vi "DrivePropertiesConvert.vi"(4 "Position Offset In":dbl, 5 "Channel Properties In":T2={"Channel Name"="", "Vel. Default"=5.0, "Acc. Default"=5.0, "Vel. Max"=5.0, "Vel. Min"=5.0, "Acc. Max"=5.0, "Acc. Min"=5.0, "Pulses/unit"=0.0, "Address"=0, "Pulse Offset"=0, "Pos Tolerance"=0.0, "Pulses/rev"=0.0, "Backlash/Eng units"=0.0, "Current Pos"=0.0, "Ch Status"=enum."Active", "Port Name"="", "Axis Transform mode"="", "Metadata Ch Name"="", "Type"=enum."MCode", "De Power Motor"=enum."FALSE", "ConfigString"=""} {"Current Pos" format="%.2f"; "Backlash/Eng units" format="%.2f"; "Pulses/rev" format="%.2f"; "Pos Tolerance" format="%.2f"; "Pulses/unit" format="%.2f"; "Acc. Min" format="%.2f"; "Acc. Max" format="%.2f"; "Vel. Min" format="%.2f"; "Vel. Max" format="%.2f"; "Acc. Default" format="%.2f"; "Vel. Default" format="%.2f"}, 6 "String in":string[](array[string]), 7 "Ch names In":string[](array[string]), 8 "Mode":enum16{"Cluster to String", "String to Cluster"}(ring)) -> (0 "Channel Properties Out":T2={"Channel Name"="", "Vel. Default"=5.0, "Acc. Default"=5.0, "Vel. Max"=5.0, "Vel. Min"=5.0, "Acc. Max"=5.0, "Acc. Min"=5.0, "Pulses/unit"=0.0, "Address"=0, "Pulse Offset"=0, "Pos Tolerance"=0.0, "Pulses/rev"=0.0, "Backlash/Eng units"=0.0, "Current Pos"=0.0, "Ch Status"=enum."Active", "Port Name"="", "Axis Transform mode"="", "Metadata Ch Name"="", "Type"=enum."MCode", "De Power Motor"=enum."FALSE", "ConfigString"=""} {"Current Pos" format="%.2f"; "Backlash/Eng units" format="%.2f"; "Pulses/rev" format="%.2f"; "Pos Tolerance" format="%.2f"; "Pulses/unit" format="%.2f"; "Acc. Min" format="%.2f"; "Acc. Max" format="%.2f"; "Vel. Min" format="%.2f"; "Vel. Max" format="%.2f"; "Acc. Default" format="%.2f"; "Vel. Default" format="%.2f"}, 1 "String Values":string[](array[string]), 2 "Ch names":string[](array[string]), 3 "Position Offset Out":dbl)   [LabVIEW 2022 SP3]
uses:
  DriveProperties.ctl
  Traverse Type.ctl
panel:
  in  "Type":T1
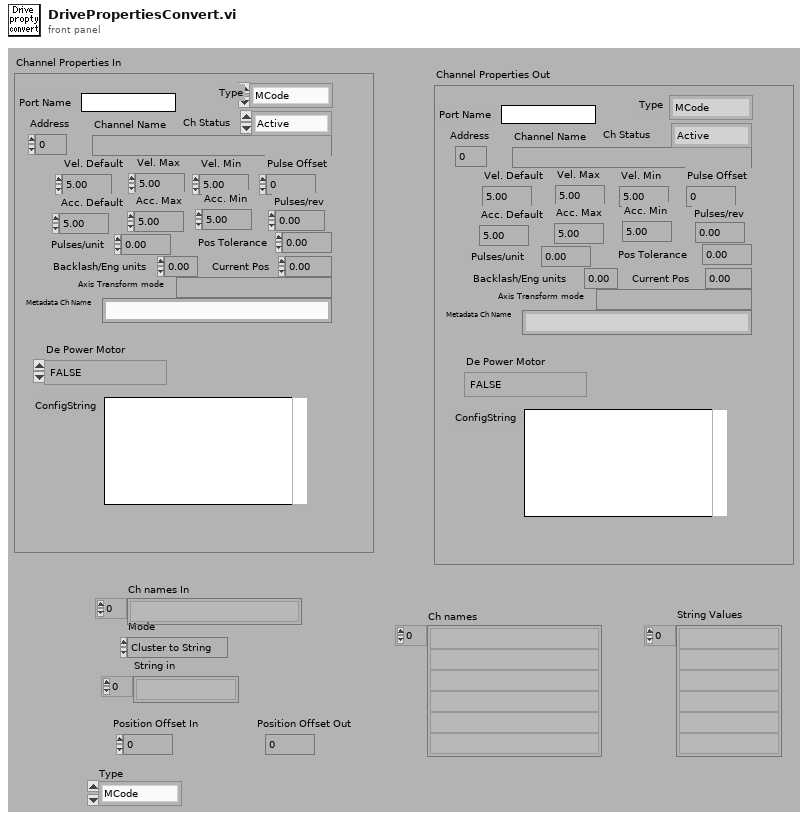
[diagram p1: front panel]
types:
  T1 = typedef "Traverse Type.ctl" = enum16{"MCode", "Dynamixel"}
  T2 = typedef "DriveProperties.ctl" = cluster{"Channel Name":string, "Vel. Default":sgl, "Acc. Default":sgl, "Vel. Max":sgl, "Vel. Min":sgl, "Acc. Max":sgl, "Acc. Min":sgl, "Pulses/unit":sgl, "Address":u8, "Pulse Offset":i32, "Pos Tolerance":sgl, "Pulses/rev":sgl, "Backlash/Eng units":sgl, "Current Pos":sgl, "Ch Status":enum16{"Active", "Offline", "Simulate"}, "Port Name":string, "Axis Transform mode":string, "Metadata Ch Name":string, "Type":T1, "De Power Motor":enum16{"TRUE", "FALSE"}, "ConfigString":string}
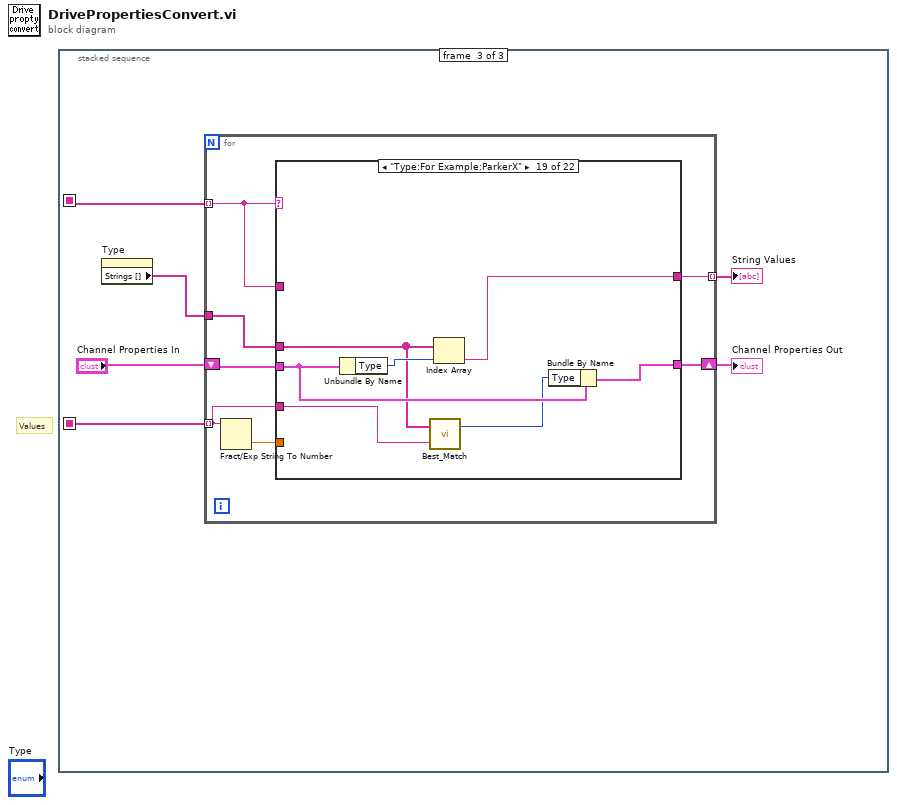
[diagram p0: block diagram]
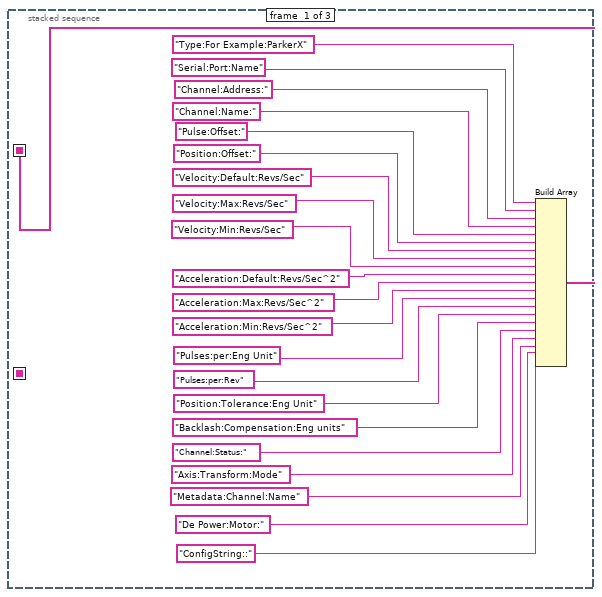
[diagram p2: hidden frame]
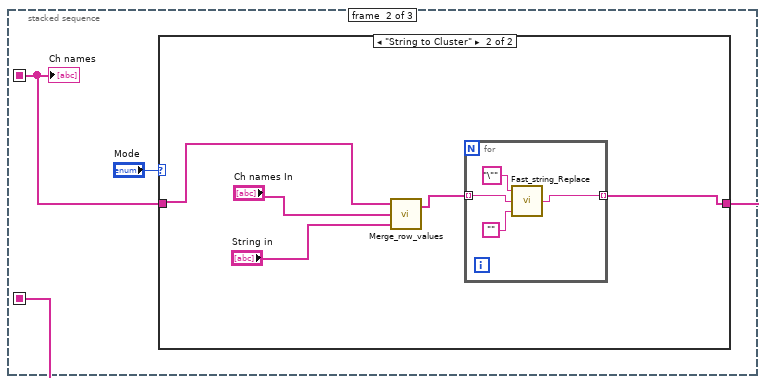
[diagram p3: hidden frame]
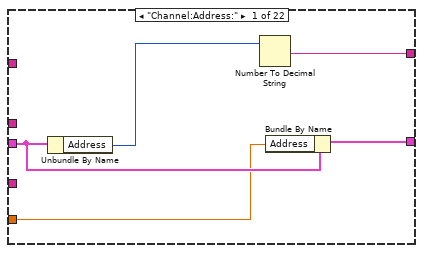
[diagram p5: hidden frame]
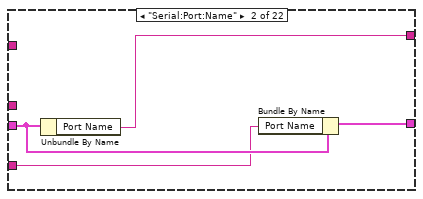
[diagram p6: hidden frame]
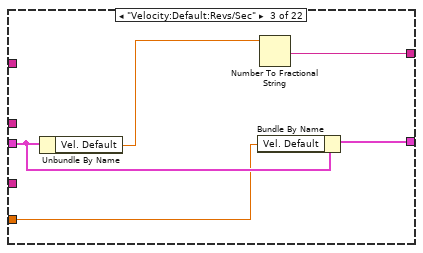
[diagram p7: hidden frame]
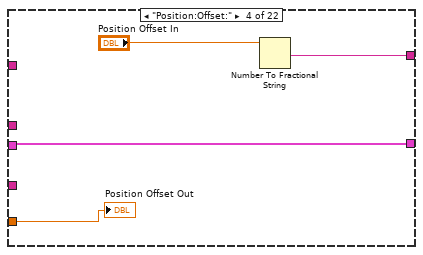
[diagram p8: hidden frame]
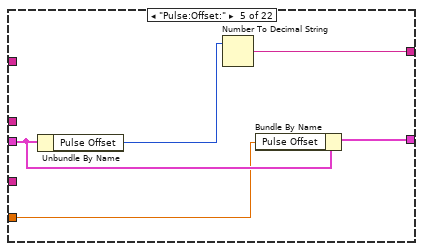
[diagram p9: hidden frame]
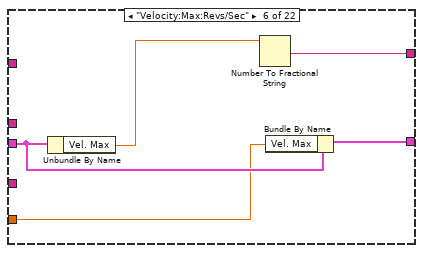
[diagram p10: hidden frame]
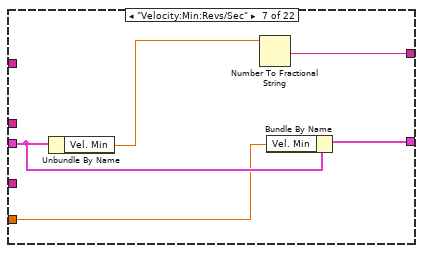
[diagram p11: hidden frame]
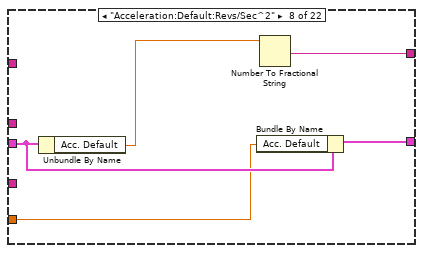
[diagram p12: hidden frame]
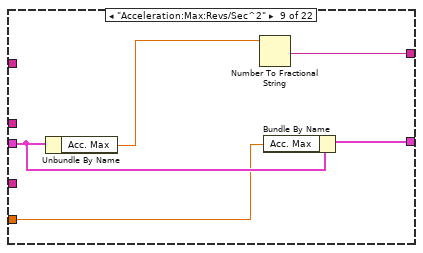
[diagram p13: hidden frame]
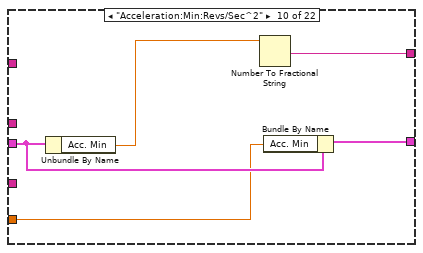
[diagram p14: hidden frame]
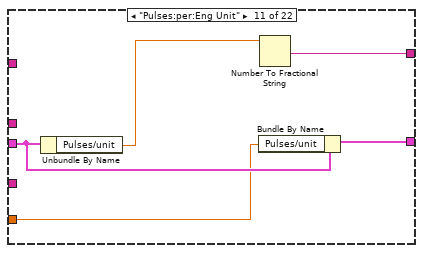
[diagram p15: hidden frame]
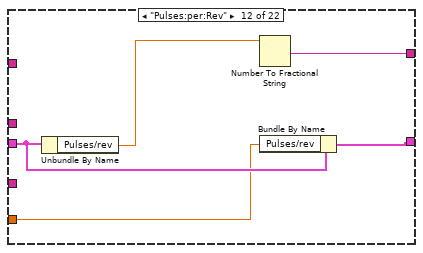
[diagram p16: hidden frame]
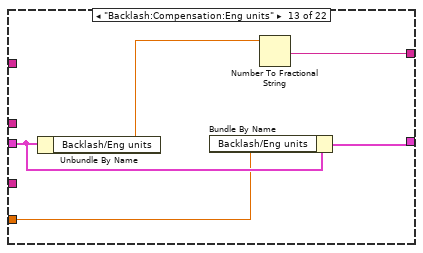
[diagram p17: hidden frame]
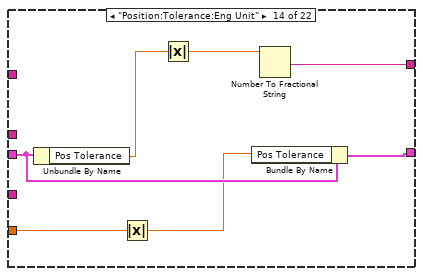
[diagram p18: hidden frame]
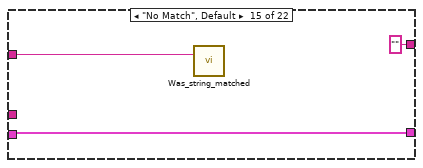
[diagram p19: hidden frame]
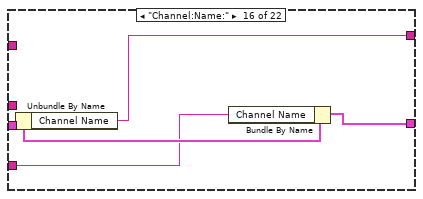
[diagram p20: hidden frame]
diagram:
  # "Values"
  n1 = stacked-sequence {
    seq-local: [w13 _ _] -> [_ w24 w41]
    seq-local: [_ w23 _] -> [_ _ w40]
    frame #0 {
      n2 = Build Array("Type:For Example:ParkerX", "Serial:Port:Name", "Channel:Address:", "Channel:Name:", "Pulse:Offset:", "Position:Offset:", "Velocity:Default:Revs/Sec", "Velocity:Max:Revs/Sec", "Velocity:Min:Revs/Sec", "Acceleration:Default:Revs/Sec^2", "Acceleration:Max:Revs/Sec^2", "Acceleration:Min:Revs/Sec^2", "Pulses:per:Eng Unit", "Pulses:per:Rev", "Position:Tolerance:Eng Unit", "Backlash:Compensation:Eng units", "Channel:Status:", "Axis:Transform:Mode", "Metadata:Channel:Name", "De Power:Motor:", "ConfigString::") -> (w13:string[])
    }
    frame #1 {
      n3 = case shown="\"String to Cluster\"" "Mode" {
        tunnel: [w26 w27] -> w23
        tunnel: w24 -> [w26 w29]
        frame "Cluster to String" {
        }
        frame "String to Cluster" {
          n4 = call "Merge_row_values.vi"("Present Row values"="String in", "Present Channels"="Ch names In", "Desired Channels"=w29) -> ("Desired Row values"=w28:string[])  [unwired: 1 out]
          n5 = for {
            tunnel: w28 -> [w35] mode=indexing
            tunnel: [w34] -> w27 mode=indexing
            n6 = call "Fast_string_Replace.vi"("Replace match with:"="", "Input String"=w35, "matchThis"="\"" ("regular expression")) -> ("Output String"=w34:string)  [unwired: 1 in, 1 out]
          }
        }
      }
      "Ch names" <- w24
    }
    frame #2 {
      n7 = property on="Type" class="Enum (strict)"() -> ("Strings []"=w36:string[])  [unwired: 2 in, 2 out]
      n8 = for {
        tunnel: w41 -> [w45] mode=indexing
        tunnel: w40 -> [w48] mode=indexing
        tunnel: [w46] -> w39 mode=indexing
        shift-right: [w43] -> w37
        shift-left: "Channel Properties In" -> [w44]
        tunnel: w36 -> [w42]
        n9 = Fract/Exp String To Number(string=w48) -> (number=w47:dbl)  [unwired: 4 out]
        n10 = case shown="\"Type:For Example:ParkerX\"" w45 {
          tunnel: w44 -> [w53 w57 w62 w64 w71 w76 w81 w86 w91 w96 w101 w106 w111 w118 w119 w124 w128 w132 w140 w146 w161 w171]
          tunnel: w48 -> [_ w55 _ _ _ _ _ _ _ _ _ _ _ _ _ w123 w127 w131 w136 w142 w157 w166]
          tunnel: [w50 w56 w59 w66 w67 w73 w78 w83 w88 w93 w98 w103 w108 w115 "" ("Channel Name") w125 w129 w133 w137 w143 w155 w168] -> w46
          tunnel: w47 -> [w52 _ w61 w63 w70 w75 w80 w85 w90 w95 w100 w105 w110 w117 _ _ _ _ _ _ _ _]
          tunnel: w45 -> [_ _ _ _ _ _ _ _ _ _ _ _ _ _ w120 _ _ _ _ _ _ _]
          tunnel: [w49 w54 w58 w64 w69 w72 w77 w82 w87 w92 w97 w102 w107 w112 w119 w122 w126 w130 w139 w145 w160 w170] -> w43
          tunnel: w42 -> [_ _ _ _ _ _ _ _ _ _ _ _ _ _ _ _ _ _ w135 _ _ _]
          frame "Channel:Address:" {
            n11 = Unbundle By Name(w53) -> ("Address"=w51:u8)
            n12 = Number To Decimal String(number=w51) -> (decimal integer string=w50:string)  [unwired: 1 out]
            n13 = Bundle By Name(cluster=w53, "Address"=w52) -> (w49:T2)
          }
          frame "Serial:Port:Name" {
            n14 = Unbundle By Name(w57) -> ("Port Name"=w56:string)
            n15 = Bundle By Name(cluster=w57, "Port Name"=w55) -> (w54:T2)
          }
          frame "Velocity:Default:Revs/Sec" {
            n16 = Unbundle By Name(w62) -> ("Vel. Default"=w60:sgl)
            n17 = Bundle By Name(cluster=w62, "Vel. Default"=w61) -> (w58:T2)
            n18 = Number To Fractional String(number=w60) -> (F-format string=w59:string)  [unwired: 3 out]
          }
          frame "Position:Offset:" {
            n19 = Number To Fractional String(number="Position Offset In") -> (F-format string=w66:string)  [unwired: 3 out]
            "Position Offset Out" <- w63
          }
          frame "Pulse:Offset:" {
            n20 = Unbundle By Name(w71) -> ("Pulse Offset"=w68:i32)
            n21 = Number To Decimal String(number=w68) -> (decimal integer string=w67:string)  [unwired: 1 out]
            n22 = Bundle By Name(cluster=w71, "Pulse Offset"=w70) -> (w69:T2)
          }
          frame "Velocity:Max:Revs/Sec" {
            n23 = Unbundle By Name(w76) -> ("Vel. Max"=w74:sgl)
            n24 = Number To Fractional String(number=w74) -> (F-format string=w73:string)  [unwired: 3 out]
            n25 = Bundle By Name(cluster=w76, "Vel. Max"=w75) -> (w72:T2)
          }
          frame "Velocity:Min:Revs/Sec" {
            n26 = Unbundle By Name(w81) -> ("Vel. Min"=w79:sgl)
            n27 = Number To Fractional String(number=w79) -> (F-format string=w78:string)  [unwired: 3 out]
            n28 = Bundle By Name(cluster=w81, "Vel. Min"=w80) -> (w77:T2)
          }
          frame "Acceleration:Default:Revs/Sec^2" {
            n29 = Unbundle By Name(w86) -> ("Acc. Default"=w84:sgl)
            n30 = Bundle By Name(cluster=w86, "Acc. Default"=w85) -> (w82:T2)
            n31 = Number To Fractional String(number=w84) -> (F-format string=w83:string)  [unwired: 3 out]
          }
          frame "Acceleration:Max:Revs/Sec^2" {
            n32 = Unbundle By Name(w91) -> ("Acc. Max"=w89:sgl)
            n33 = Number To Fractional String(number=w89) -> (F-format string=w88:string)  [unwired: 3 out]
            n34 = Bundle By Name(cluster=w91, "Acc. Max"=w90) -> (w87:T2)
          }
          frame "Acceleration:Min:Revs/Sec^2" {
            n35 = Unbundle By Name(w96) -> ("Acc. Min"=w94:sgl)
            n36 = Number To Fractional String(number=w94) -> (F-format string=w93:string)  [unwired: 3 out]
            n37 = Bundle By Name(cluster=w96, "Acc. Min"=w95) -> (w92:T2)
          }
          frame "Pulses:per:Eng Unit" {
            n38 = Unbundle By Name(w101) -> ("Pulses/unit"=w99:sgl)
            n39 = Bundle By Name(cluster=w101, "Pulses/unit"=w100) -> (w97:T2)
            n40 = Number To Fractional String(number=w99) -> (F-format string=w98:string)  [unwired: 3 out]
          }
          frame "Pulses:per:Rev" {
            n41 = Unbundle By Name(w106) -> ("Pulses/rev"=w104:sgl)
            n42 = Number To Fractional String(number=w104) -> (F-format string=w103:string)  [unwired: 3 out]
            n43 = Bundle By Name(cluster=w106, "Pulses/rev"=w105) -> (w102:T2)
          }
          frame "Backlash:Compensation:Eng units" {
            n44 = Unbundle By Name(w111) -> ("Backlash/Eng units"=w109:sgl)
            n45 = Bundle By Name(cluster=w111, "Backlash/Eng units"=w110) -> (w107:T2)
            n46 = Number To Fractional String(number=w109) -> (F-format string=w108:string)  [unwired: 3 out]
          }
          frame "Position:Tolerance:Eng Unit" {
            n47 = Unbundle By Name(w118) -> ("Pos Tolerance"=w116:sgl)
            n48 = Absolute Value(x=w117) -> (abs(x)=w113:dbl)
            n49 = Absolute Value(x=w116) -> (abs(x)=w114:sgl)
            n50 = Bundle By Name(cluster=w118, "Pos Tolerance"=w113) -> (w112:T2)
            n51 = Number To Fractional String(number=w114) -> (F-format string=w115:string)  [unwired: 3 out]
          }
          frame "No Match", Default {
            n52 = call "Was_string_matched.vi"("Variable name"=w120) -> ()  [unwired: 2 in]
          }
          frame "Channel:Name:" {
            n53 = Unbundle By Name(w124) -> ("Channel Name"=w125:string)
            n54 = Bundle By Name(cluster=w124, "Channel Name"=w123) -> (w122:T2)
          }
          frame "Axis:Transform:Mode" {
            n55 = Unbundle By Name(w128) -> ("Axis Transform mode"=w129:string)
            n56 = Bundle By Name(cluster=w128, "Axis Transform mode"=w127) -> (w126:T2)
          }
          frame "Metadata:Channel:Name" {
            n57 = Unbundle By Name(w132) -> ("Metadata Ch Name"=w133:string)
            n58 = Bundle By Name(cluster=w132, "Metadata Ch Name"=w131) -> (w130:T2)
          }
          frame "Type:For Example:ParkerX" {
            n59 = Unbundle By Name(w140) -> ("Type"=w138:T1)
            n60 = call "Best_Match.vi"("Input String"=w136, "String Options"=w135) -> ("index of element"=w134:i32)  [unwired: 1 out]
            n61 = Index Array(array=w135, index=w138) -> (element=w137:string)
            n62 = Bundle By Name(cluster=w140, "Type"=w134) -> (w139:T2)
          }
          frame "Channel:Status:" {
            n63 = Unbundle By Name(w146) -> ("Ch Status"=w144:enum16{"Active", "Offline", "Simulate"})
            n64 = case shown="\"Active\"" w144 {
              tunnel: ["Active" "Simulate" "Offline"] -> w143
              frame "Active" {
              }
              frame "Simulate" {
              }
              frame "Offline" {
              }
            }
            n65 = case shown="\"Active\", Default" w142 {
              tunnel: [enum16{"Active", "Offline", "Simulate"}."Active" ("Ch Status") enum16{"Active", "Offline", "Simulate"}."Simulate" ("Ch Status") enum16{"Active", "Offline", "Simulate"}."Offline" ("Ch Status") enum16{"Active", "Offline", "Simulate"}."Active" ("Ch Status") enum16{"Active", "Offline", "Simulate"}."Offline" ("Ch Status")] -> w141
              frame "Active", Default {
              }
              frame "Simulate" {
              }
              frame "Offline" {
              }
              frame "TRUE" {
              }
              frame "FALSE" {
              }
            }
            n66 = Bundle By Name(cluster=w146, "Ch Status"=w141) -> (w145:T2)
          }
          frame "ConfigString::" {
            n67 = Unbundle By Name(w161) -> ("ConfigString"=w155:string)
            n68 = Empty String/Path?(string/path=w157) -> (empty?=w158:bool)
            n69 = Select(t="Not Used", s=w158, f=w157) -> (s? t:f=w156:string)
            n70 = Bundle By Name(cluster=w161, "ConfigString"=w156) -> (w160:T2)
          }
          frame "De Power:Motor:" {
            w169 = string[] ["TRUE", "FALSE"] ("Read Attribute")
            n71 = Unbundle By Name(w171) -> ("De Power Motor"=w167:enum16{"TRUE", "FALSE"})
            n72 = Search 1D Array(1D array=w169, element=w166) -> (index of element=w163:i32)  [unwired: 1 out]
            n73 = Index Array(array=w169, index=w167) -> (element=w168:string)
            n74 = Less Than 0?(x=w163) -> (x < 0?=w165:bool)
            n75 = Select(t=0, s=w165, f=w163) -> (s? t:f=w162:i32)
            n76 = Bundle By Name(cluster=w171, "De Power Motor"=w162) -> (w170:T2)
          }
        }
      }
      "Channel Properties Out" <- w37
      "String Values" <- w39
    }
  }
